vi "Create Channel Task.vi"(8 "error in":errorcluster, 10 "SQL query":string="SELECT max(MaximumVoltage),max(MinimumVoltage), max(TerminalConfiguration),max(SampleRate) FROM\nltt.daq_configuration \nWhere ChannelType='Analog_Input' and Enabled=1;", 11 "NI Analog Input in":refnum<class "NI Analog Input.lvclass">) -> (0 "error out":errorcluster, 3 "NI Analog Input out":refnum<class "NI Analog Input.lvclass">)   [LabVIEW 2023, in "HardwareAbstractionLayer_LVOOP.lvlib" / "NI Analog Input.lvclass"]
doc: "This VI Analog Input Voltage Created the Task Physical Channel"
uses:
  NI Analog Input.lvclass
  NI Analog Input.lvclass/NI Analog Input.ctl
  <vilib>/DAQmx/create/channels.llb/DAQmx Create Channel (AI-Voltage-Basic).vi
  <vilib>/DAQmx/configure/timing.llb/DAQmx Timing (Sample Clock).vi
  Database/Database.lvclass
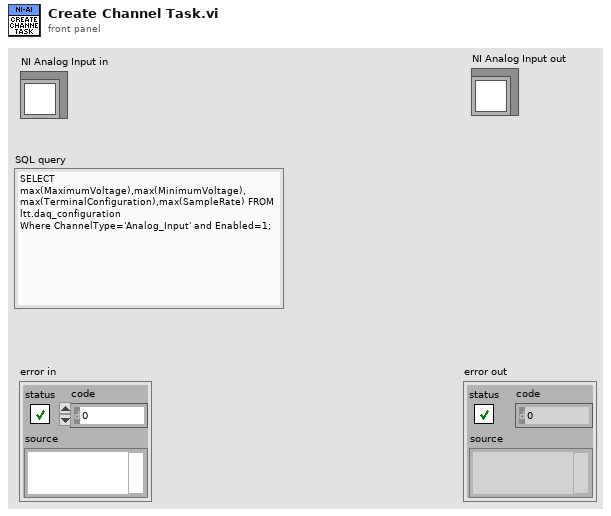
[diagram p1: front panel]
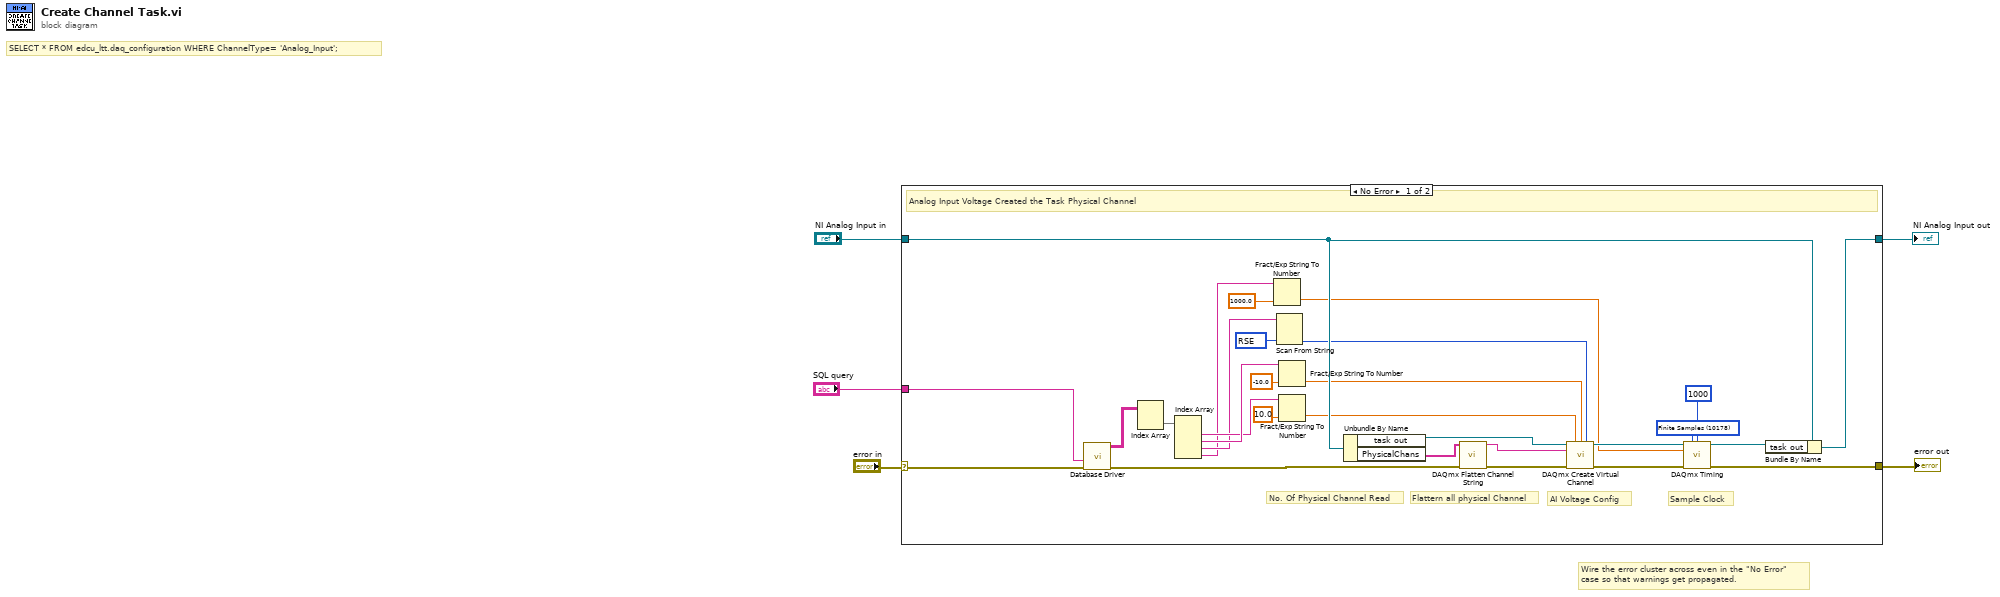
[diagram p0: block diagram]
diagram:
  # "Wire the error cluster across even in the \"No Error\"\ncase so that warnings get propagated."
  # "SELECT * FROM edcu_ltt.daq_configuration WHERE ChannelType= 'Analog_Input';"
  n1 = case shown="No Error" "error in" {
    selector: "error in" -> [w16 w36]
    tunnel: [w11 w36] -> w4
    tunnel: [w33 w35] -> w2
    tunnel: "NI Analog Input in" -> [w34 w35]
    tunnel: "SQL query" -> [w10 _]
    frame No Error {
      w8 = 10178 items=["Finite Samples"=10178, "Continuous Samples"=10123, "Hardware Timed Single Point"=12522] ("sample mode")
      w29 = 10083 items=["Default"=-1, "RSE"=10083, "NRSE"=10078, "Differential"=10106, "Pseudodifferential"=12529] ("input terminal configuration")
      # "Sample Clock"
      # "AI Voltage Config"
      # "Flattern all physical Channel"
      # "No. Of Physical Channel Read"
      # "Analog Input Voltage Created the Task Physical Channel"
      n2 = call "Database Driver.vi"("error in"=w16, "SQL query"=w10) -> ("error out"=w15:errorcluster, "data"=w14:string[][])  [unwired: 6 in, 2 out]
      n3 = Index Array(array=w14) -> (element=w30:string[])  [unwired: 2 in]
      n4 = Index Array(array=w30) -> (element #1=w31:string, element #2=w32:string, element #3=w23:string, element #4=w18:string)  [unwired: 4 in]
      n5 = Fract/Exp String To Number(string=w18, default (0 dbl)=1000.0 ("rate")) -> (number=w6:dbl)  [unwired: 2 in, 1 out]
      n6 = Scan From String(input string=w23, default 1=w29) -> (output 1=w24:i32)  [unwired: 3 in, 3 out]
      n7 = Fract/Exp String To Number(string=w32, default (0 dbl)=-10.0 ("maximum value")) -> (number=w25:dbl)  [unwired: 2 in, 1 out]
      n8 = Fract/Exp String To Number(string=w31, default (0 dbl)=10.0 ("maximum value")) -> (number=w26:dbl)  [unwired: 2 in, 1 out]
      n9 = Unbundle By Name(w34) -> ("task out"=w21:refnum<k21>, "PhysicalChans"=w13:tag[])
      n10 = call <vilib>:"DAQmx Flatten Channel String.vi"("names in"=w13, "error in"=w15) -> ("names out"=w12:string, "error out"=w22:errorcluster)  [unwired: 12 in]
      n11 = call-poly <vilib>:"DAQmx Create Virtual Channel.vi"("task in"=w21, "maximum value"=w26, "minimum value"=w25, "input terminal configuration"=w24, "physical channels"=w12, "error in"=w22) -> ("task out"=w9:refnum<k21>, "error out"=w20:errorcluster)  [unwired: 8 in]
      n12 = call-poly <vilib>:"DAQmx Timing.vi"("task/channels in"=w9, "sample mode"=w8, "samples per channel"=1000, "rate"=w6, "error in"=w20) -> ("task out"=w17:refnum<k21>, "error out"=w11:errorcluster)  [unwired: 9 in]
      n13 = Bundle By Name(cluster=w34, "task out"=w17) -> (w33:refnum<class "NI Analog Input.lvclass">)
    }
    frame Error {
    }
  }
  "error out" <- w4
  "NI Analog Input out" <- w2
